vi "Read CSV.vi"(8 "error in (no error)":errorcluster, 11 "Path":path) -> (0 "error out":errorcluster, 2 "first row":dbl[](array[numeric]) format="%0.3f", 3 "all rows":dbl[][](array[numeric]) format="%0.3f")   [LabVIEW 2014, in "AvaSpec.lvlib"]
uses:
  AvaSpec.lvlib
  <vilib>/Utility/file.llb/Read From Spreadsheet File (DBL).vi
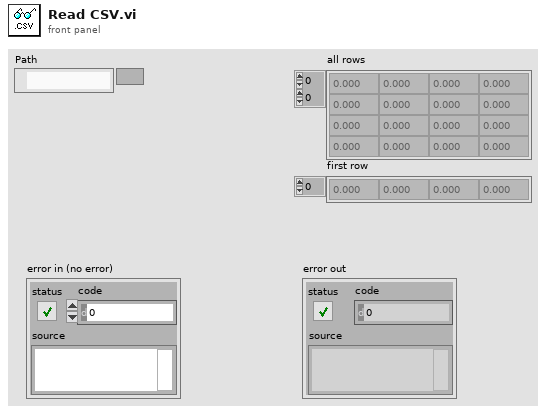
[diagram p1: front panel]
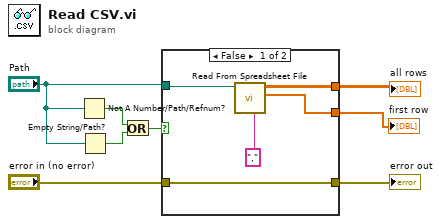
[diagram p0: block diagram]
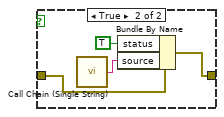
[diagram p2: hidden frame]
diagram:
  n1 = Not A Number/Path/Refnum?(number/path/refnum="Path") -> (NaN/Path/Refnum?=w8:bool)
  n2 = Empty String/Path?(string/path="Path") -> (empty?=w7:bool)
  n3 = Or(x=w8, y=w7) -> (x .or. y?=w6:bool)
  n4 = case shown="False" w6 {
    tunnel: "error in (no error)" -> [w12 w17]
    tunnel: [w12 w14] -> w4
    tunnel: [w11 _] -> w3
    tunnel: [w10 _] -> w2
    tunnel: "Path" -> [w9 _]
    frame False {
      n5 = call-poly <vilib>:"Read From Spreadsheet File.vi"("delimiter (\\t)"="," ("delimiter (\\t)"), "file path (dialog if empty)"=w9) -> ("first row"=w10:dbl[], "all rows"=w11:dbl[][])  [unwired: 5 in, 3 out]
    }
    frame True {
      n6 = call "Call Chain (Single String).vi"() -> ("Call Chain"=w15:string)
      n7 = Bundle By Name(cluster=w17, "status"=TRUE, "source"=w15) -> (w14:errorcluster)
    }
  }
  "error out" <- w4
  "all rows" <- w3
  "first row" <- w2
